vi "_Object Tester.vi"() -> ()   [LabVIEW 2025, in "Motor.lvlib" / "Stepper.lvclass"]
uses:
  Stepper.lvclass
  Motor Selection.ctl
  USB IO/Classes/USB-6000/USB-6000.lvclass
  CL57RS/CL57RS.lvclass
  C:/Users/Tyson.Grover/Desktop/Repositories/dqmh-lvoop-template/Libraries/Motor/Classes/Stepper/Stepper.lvclass
  <vilib>/Handler Framework/CmdQueue/Enqueue Single.vi
  Stepper.lvclass/Stepper.ctl
  <vilib>/Handler Framework/Handler Framework.lvlib
  C:/Users/Tyson.Grover/Desktop/Repositories/dqmh-lvoop-template/Libraries/Motor/Classes/CL57RS/CL57RS.lvclass
panel:
  out "error out":errorcluster
  in  "Tab Control":enum32{"JOG", "Adjust Param"}(tab)
  in  "Motor Brake":bool
  in  "Clear Motor Error":bool
  in  "CCW?":bool
  in  "JOG":bool
  in  "Speed [rpm]":dbl(slide)=9.818181818181818 min=0.0 max=100.0 scale=0.0..100.0
  in  "Angle":dbl(knob) scale=-180.0..180.0
  in  "Go To Angle":bool
  out "Value of Reading":u16 format="%.0x"
  in  "Register 2":u16 format="%.0x"
  in  "Value":u16
  in  "Register":u16 format="%.0x"
  in  "Adjust Register":bool
  out "Value of Reading 2":u16 format="%.0b"
  out "Value of Reading 3":u16
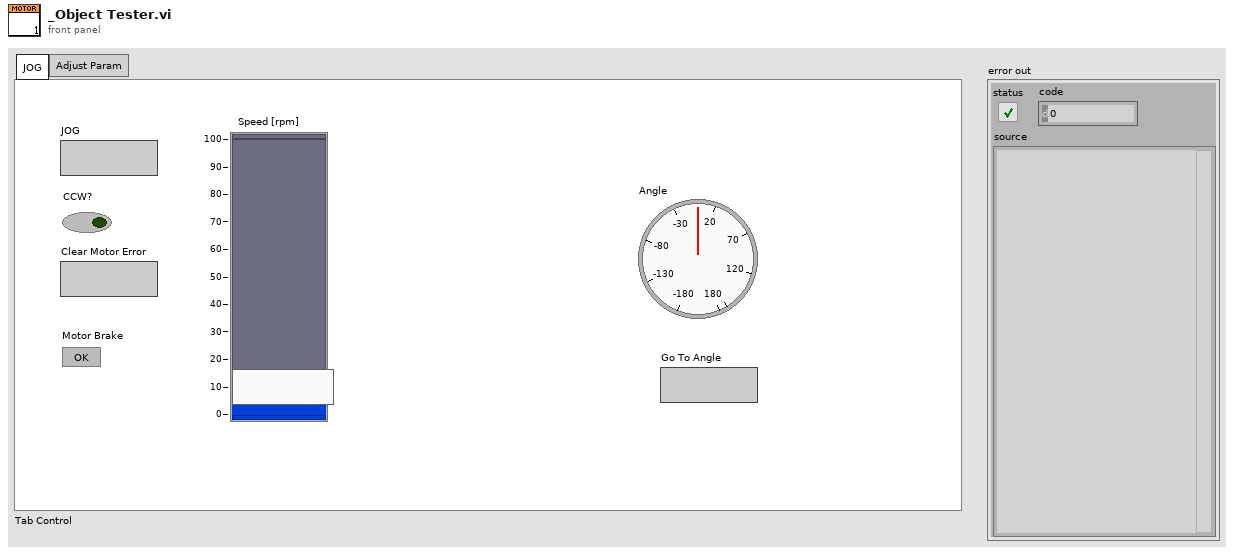
[diagram p1: front panel]
types:
  T1 = typedef "Motor Selection.ctl" = enum16{"Stepper", "CL57RS"}
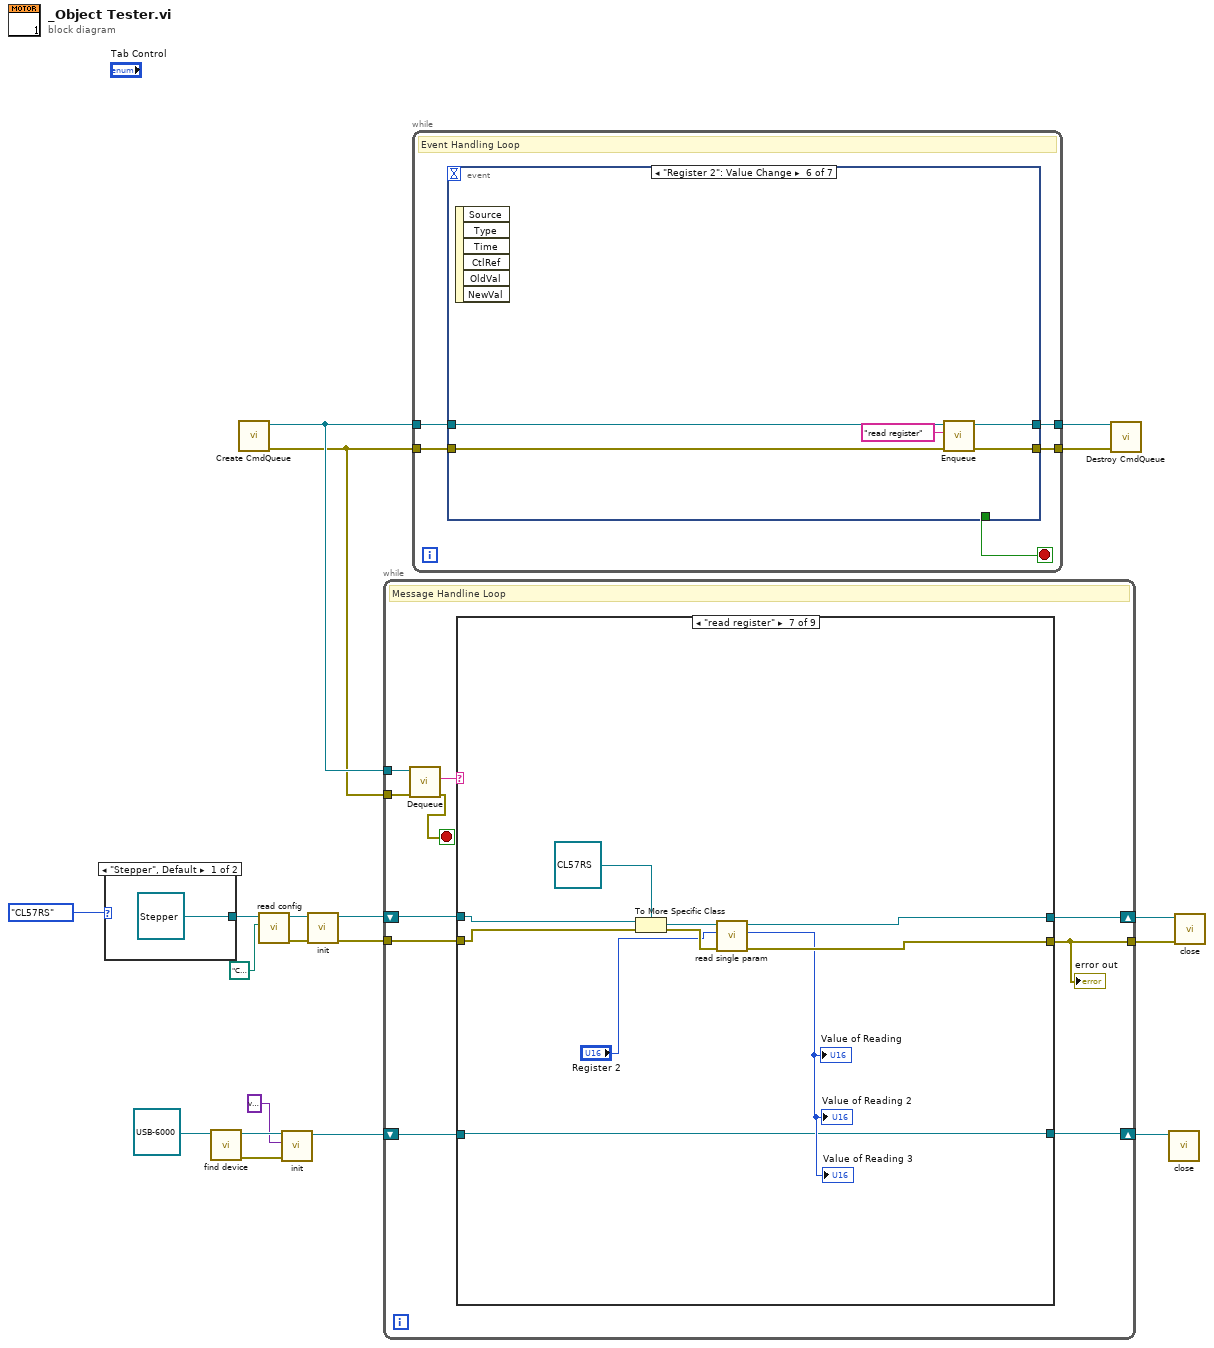
[diagram p0: block diagram]
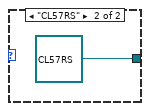
[diagram p2: hidden frame]
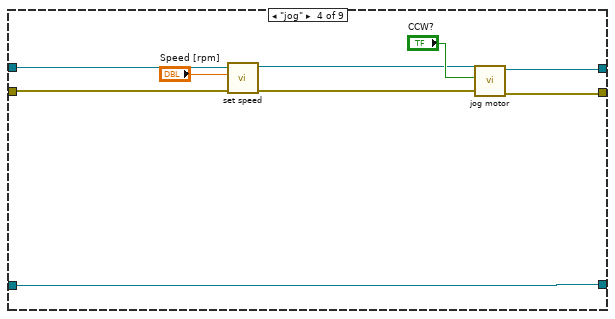
[diagram p6: hidden frame]
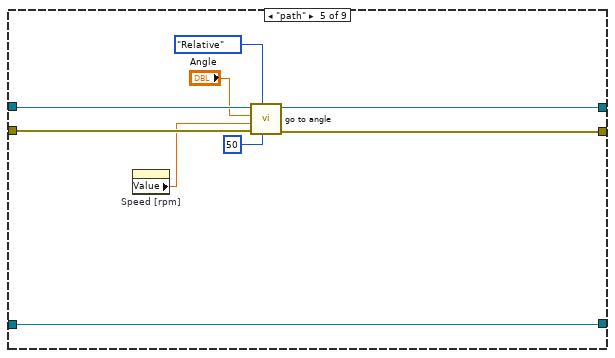
[diagram p7: hidden frame]
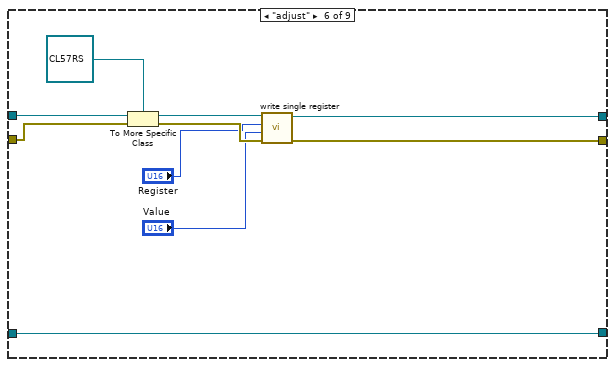
[diagram p8: hidden frame]
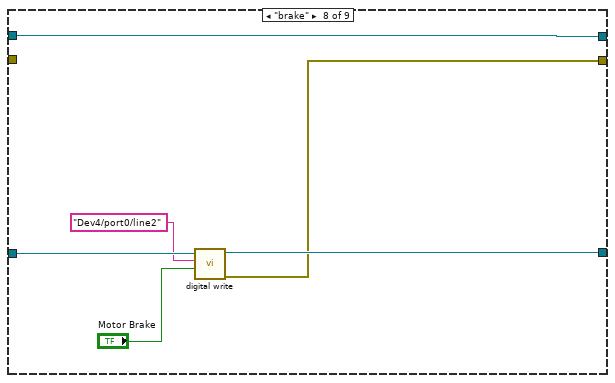
[diagram p9: hidden frame]
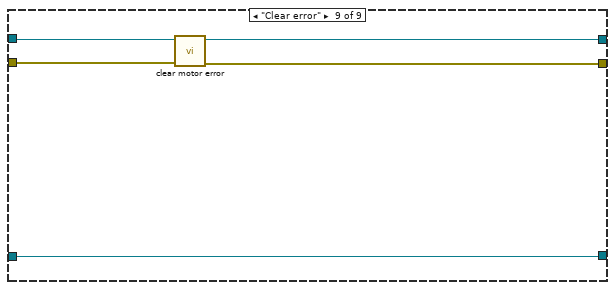
[diagram p10: hidden frame]
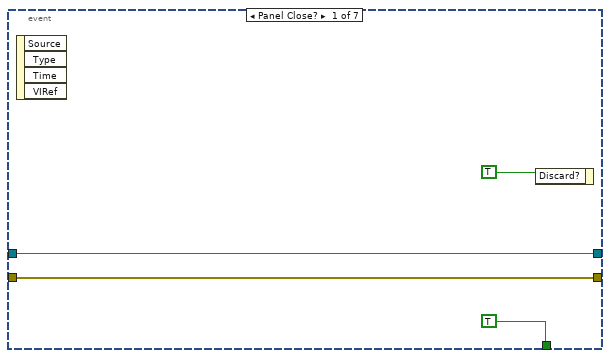
[diagram p11: hidden frame]
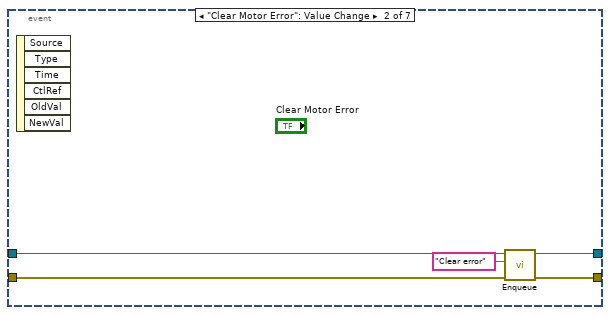
[diagram p12: hidden frame]
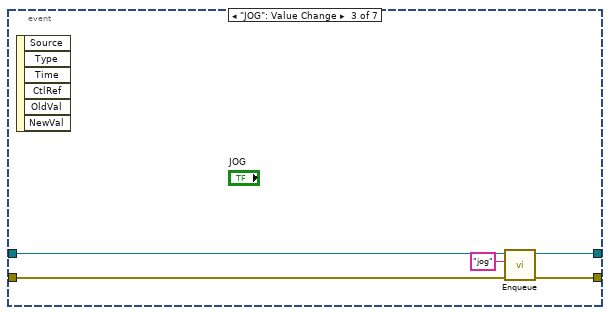
[diagram p13: hidden frame]
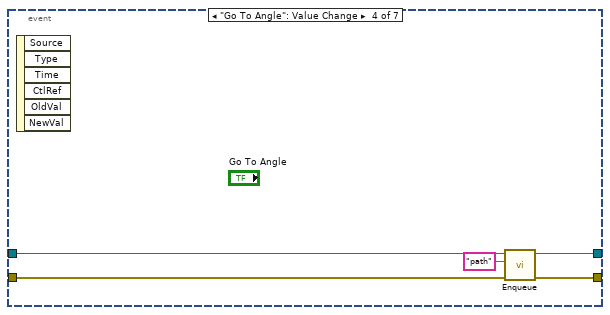
[diagram p14: hidden frame]
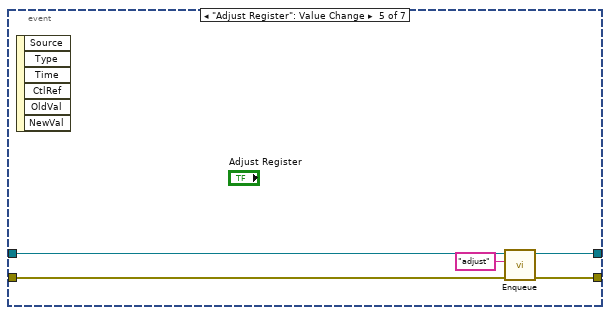
[diagram p15: hidden frame]
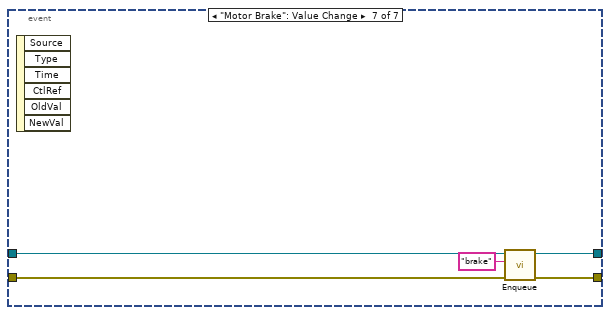
[diagram p16: hidden frame]
diagram:
  n1 = case shown="\"Stepper\", Default" Motor_Selection."CL57RS" {
    tunnel: [refnum<class "Stepper.lvclass"> refnum ("Motor.lvlib:Stepper.lvclass") refnum<class "CL57RS.lvclass"> refnum ("Motor.lvlib:CL57RS.lvclass")] -> w14
    frame "Stepper", Default {
    }
    frame "CL57RS" {
    }
  }
  n2 = call-dynamic "find device.vi"("USB-6000 in"=refnum<class "USB-6000.lvclass"> refnum ("USB IO.lvlib:USB-6000.lvclass")) -> ("error out"=w3:errorcluster, "USB-6000 out"=w5:refnum<class "USB-6000.lvclass">)  [unwired: 9 in]
  n3 = call <vilib>:"Create CmdQueue.vi"() -> ("error out"=w18:errorcluster, "CmdQueue out"=w19:refnum<queue>)  [unwired: 10 in]
  n4 = call-dynamic "read config.vi"("Config File Path"=path "C:/Users/Tyson.Grover/Desktop/Repositories/dqmh-lvoop-template/Config/dqmh-lvoop-template/motor-config.json", "Stepper in"=w14) -> ("error out"=w12:errorcluster, "Stepper out"=w13:refnum<class "Stepper.lvclass">)  [unwired: 8 in]
  n5 = call-dynamic "init.vi"("error in (no error)"=w3, "Variant"=variant, "USB-6000 in"=w5) -> ("USB-6000 out"=w2:refnum<class "USB-6000.lvclass">)  [unwired: 7 in, 1 out]
  n6 = call-dynamic "init.vi"("error in (no error)"=w12, "Stepper in"=w13) -> ("error out"=w9:errorcluster, "Stepper out"=w10:refnum<class "Stepper.lvclass">)  [unwired: 8 in]
  n7 = while {
    tunnel: w19 -> [w31]
    tunnel: w18 -> [w30]
    tunnel: w9 -> [w26]
    shift-right: [w25] -> w8
    shift-left: w10 -> [w27]
    tunnel: [w24] -> w7
    shift-right: [w22] -> w1
    shift-left: w2 -> [w23]
    stop <- w29 stop-if-true
    # "Message Handline Loop"
    n8 = call <vilib>:"Dequeue.vi"("error in (no error)"=w30, "CmdQueue in"=w31) -> ("error out"=w29:errorcluster, "cmd"=w28:string)  [unwired: 5 in, 3 out]
    n9 = case shown="\"read register\"" w28 {
      tunnel: w27 -> [w33 w35 w37 w43 w55 w61 w74 w81 w86]
      tunnel: w26 -> [_ _ _ w42 w54 w60 w73 _ w85]
      tunnel: [w33 w35 w37 w46 w52 w64 w69 w81 w84] -> w25
      tunnel: [_ _ _ w45 w53 w58 w68 w76 w83] -> w24
      tunnel: w23 -> [w32 w34 w36 w38 w51 w65 w66 w80 w82]
      tunnel: [w32 w34 w36 w38 w51 w65 w66 w79 w82] -> w22
      frame Default {
      }
      frame "init" {
      }
      frame "shutdown" {
      }
      frame "jog" {
        n10 = call-dynamic "set speed.vi"("error in (no error)"=w42, "Speed [rpm]"="Speed [rpm]", "Stepper in"=w43) -> ("error out"=w40:errorcluster, "Stepper out"=w41:refnum<class "Stepper.lvclass">)  [unwired: 7 in]
        n11 = call-dynamic "jog motor.vi"("error in (no error)"=w40, "CCW? (T)"="CCW?", "Stepper in"=w41) -> ("error out"=w45:errorcluster, "Stepper out"=w46:refnum<class "Stepper.lvclass">)  [unwired: 7 in]
      }
      frame "path" {
        n12 = property on="Speed [rpm]" class="Slide (strict)"() -> ("Value"=w49:dbl)  [unwired: 2 in, 2 out]
        n13 = call-dynamic "go to angle.vi"("Pause Time [ms]"=50, "Relative?"=enum16{"Relative", "Absolute"}."Relative", "error in (no error)"=w54, "Velocity [rpm]"=w49, "Angle"="Angle", "Stepper in"=w55) -> ("error out"=w53:errorcluster, "Stepper out"=w52:refnum<class "Stepper.lvclass">)  [unwired: 4 in]
      }
      frame "adjust" {
        n14 = To More Specific Class(target class=refnum<class "CL57RS.lvclass"> refnum ("Motor.lvlib:CL57RS.lvclass"), reference=w61, error in=w60) -> (specific class reference=w62:refnum<class "CL57RS.lvclass">, error out=w59:errorcluster)
        n15 = call "write single register.vi"("error in (no error)"=w59, "register to write"="Value", "address"="Register", "CL57RS in"=w62) -> ("error out"=w58:errorcluster, "CL57RS out"=w64:refnum<class "CL57RS.lvclass">)  [unwired: 6 in]
      }
      frame "read register" {
        n16 = To More Specific Class(target class=refnum<class "CL57RS.lvclass"> refnum ("Motor.lvlib:CL57RS.lvclass"), reference=w74, error in=w73) -> (specific class reference=w71:refnum<class "CL57RS.lvclass">, error out=w72:errorcluster)
        n17 = call "read single param.vi"("error in (no error)"=w72, "address"="Register 2", "CL57RS in"=w71) -> ("error out"=w68:errorcluster, "register"=→"Value of Reading" →"Value of Reading 2" →"Value of Reading 3":u16, "CL57RS out"=w69:refnum<class "CL57RS.lvclass">)  [unwired: 6 in]
      }
      frame "brake" {
        n18 = call-dynamic "digital write.vi"("On/Off"="Motor Brake", "Line"="Dev4/port0/line2", "USB-6000 in"=w80) -> ("error out"=w76:errorcluster, "USB-6000 out"=w79:refnum<class "USB-6000.lvclass">)  [unwired: 7 in]
      }
      frame "Clear error" {
        n19 = call-dynamic "clear motor error.vi"("error in (no error)"=w85, "Stepper in"=w86) -> ("error out"=w83:errorcluster, "Stepper out"=w84:refnum<class "Stepper.lvclass">)  [unwired: 8 in]
      }
    }
    "error out" <- w24
  }
  n20 = while {
    tunnel: w19 -> [w90]
    tunnel: w18 -> [w89]
    tunnel: [w88] -> w17
    tunnel: [w87] -> w16
    stop <- w91 stop-if-true
    # "Event Handling Loop"
    n21 = event shown="[5] \"Register 2\": Value Change" {
      selector: _ -> [_ _ _ _ _ _ _]
      dyn-events: _ -> [_ _ _ _ _ _ _]
      timeout: _ -> [_ _ _ _ _ _ _]
      tunnel: [TRUE _ _ _ _ _ _] -> w91
      tunnel: w90 -> [w93 w97 w102 w107 w112 w117 w122]
      tunnel: w89 -> [w92 w98 w103 w108 w113 w118 w123]
      tunnel: [w93 w100 w105 w110 w115 w120 w125] -> w88
      tunnel: [w92 w99 w104 w109 w114 w119 w124] -> w87
      event Panel Close? {
        n22 = event-data() -> ()  [unwired: 1 in, 4 out]
        n23 = event-data("Discard?"=TRUE) -> ()  [unwired: 1 in, 1 out]
      }
      event "Clear Motor Error": Value Change {
        n24 = event-data() -> ()  [unwired: 1 in, 6 out]
        n25 = call-poly <vilib>:"Enqueue.vi"("error in (no error)"=w98, "Command"="Clear error", "CmdQueue in"=w97) -> ("error out"=w99:errorcluster, "CmdQueue out"=w100:refnum<queue>)  [unwired: 7 in]
      }
      event "JOG": Value Change {
        n26 = event-data() -> ()  [unwired: 1 in, 6 out]
        n27 = call-poly <vilib>:"Enqueue.vi"("error in (no error)"=w103, "Command"="jog", "CmdQueue in"=w102) -> ("error out"=w104:errorcluster, "CmdQueue out"=w105:refnum<queue>)  [unwired: 7 in]
      }
      event "Go To Angle": Value Change {
        n28 = event-data() -> ()  [unwired: 1 in, 6 out]
        n29 = call-poly <vilib>:"Enqueue.vi"("error in (no error)"=w108, "Command"="path", "CmdQueue in"=w107) -> ("error out"=w109:errorcluster, "CmdQueue out"=w110:refnum<queue>)  [unwired: 7 in]
      }
      event "Adjust Register": Value Change {
        n30 = event-data() -> ()  [unwired: 1 in, 6 out]
        n31 = call-poly <vilib>:"Enqueue.vi"("error in (no error)"=w113, "Command"="adjust", "CmdQueue in"=w112) -> ("error out"=w114:errorcluster, "CmdQueue out"=w115:refnum<queue>)  [unwired: 7 in]
      }
      event "Register 2": Value Change {
        n32 = event-data() -> ()  [unwired: 1 in, 6 out]
        n33 = call-poly <vilib>:"Enqueue.vi"("error in (no error)"=w118, "Command"="read register", "CmdQueue in"=w117) -> ("error out"=w119:errorcluster, "CmdQueue out"=w120:refnum<queue>)  [unwired: 7 in]
      }
      event "Motor Brake": Value Change {
        n34 = event-data() -> ()  [unwired: 1 in, 6 out]
        n35 = call-poly <vilib>:"Enqueue.vi"("error in (no error)"=w123, "Command"="brake", "CmdQueue in"=w122) -> ("error out"=w124:errorcluster, "CmdQueue out"=w125:refnum<queue>)  [unwired: 7 in]
      }
    }
  }
  n36 = call <vilib>:"Destroy CmdQueue.vi"("error in (no error)"=w16, "CmdQueue in"=w17) -> ()  [unwired: 9 in, 1 out]
  n37 = call-dynamic "close.vi"("USB-6000 in"=w1) -> ()  [unwired: 9 in, 2 out]
  n38 = call-dynamic "close.vi"("error in (no error)"=w7, "Stepper in"=w8) -> ()  [unwired: 8 in, 2 out]
